vi "Get Owning Path Default Value.vi"(0 "SA Path Group in":refnum<class "SA 18GHz Path Group.lvclass">, 11 "error in (no error)":errorcluster) -> (4 "SA Path Group out":refnum<class "SA 18GHz Path Group.lvclass">, 6 "Path":refnum<class "Path.lvclass">, 15 "error out":errorcluster)   [LabVIEW 2023, in "RFFixtureCharact.RFPM.lvlib" / "SA 18GHz Path Group.lvclass"]
uses:
  SA 18GHz Path Group.lvclass
  Common/Base Classes/Path/Path.lvclass
  Paths/SA Path/SA 18GHz Path.lvclass
  C:/srd-semi-rfcal-software/AuxTools/STSRFFixtureCharactUtility/Source/Code Modules/Common/Base Classes/Path/Path.lvclass
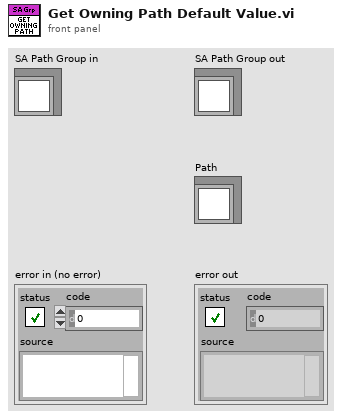
[diagram p1: front panel]
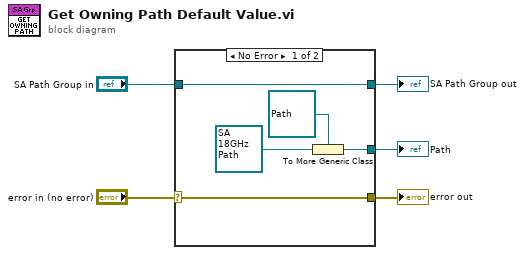
[diagram p0: block diagram]
diagram:
  n1 = case shown="No Error" "error in (no error)" {
    selector: "error in (no error)" -> [w10 w11]
    tunnel: [w6 _] -> w1
    tunnel: [w10 w11] -> w4
    tunnel: [w9 w12] -> w3
    tunnel: "SA Path Group in" -> [w9 w12]
    frame No Error {
      n2 = To More Generic Class(target class=refnum<class "Path.lvclass"> refnum ("Path"), reference=refnum<class "SA 18GHz Path.lvclass"> refnum ("STS Scalar Fixture Charact.lvlib:SA Path.lvclass")) -> (generic class reference=w6:refnum<class "Path.lvclass">)
    }
    frame Error {
    }
  }
  "error out" <- w4
  "SA Path Group out" <- w3
  "Path" <- w1
